vi "DOCK_MAIN_choose_batch_to_reload.vi"(8 "error_in":errorcluster) -> (0 "error_out":errorcluster, 1 "declared_size":u16, 2 "batch_code":string, 3 "batch_ID":string, 5 "Canceled?":bool=TRUE)   [LabVIEW 2019]
uses:
  FGV/SQL_connection/FGV_DOCK_SQL_connection.ctl
  _misc/AULocalize/SubVIs/Get Localized Phrase Compact Interface 1D.vi
  _misc/AULocalize/SubVIs/RegisterVI.vi
panel:
  in  "columns_filter":i32(listbox)
  in  "reload":bool
  in  "cancel":bool
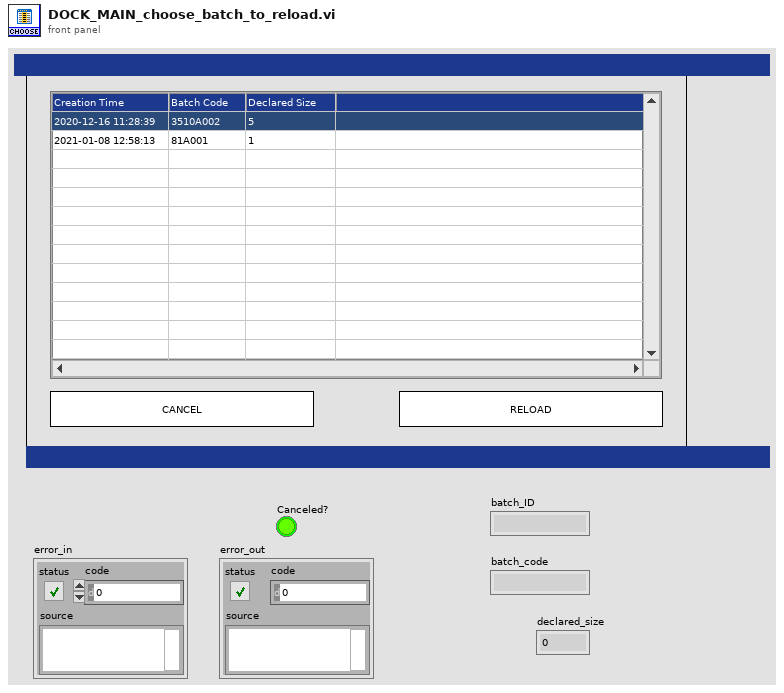
[diagram p1: front panel]
types:
  T1 = typedef "FGV_DOCK_SQL_connection.ctl" = enum16{"initialize", "connect", "read_tables", "read_columns", "SELECT", "INSERT", "UPDATE", "DELETE", "EXEC + headers", "EXEC", "TRANSACTION", "connection_active?", "disconnect"}
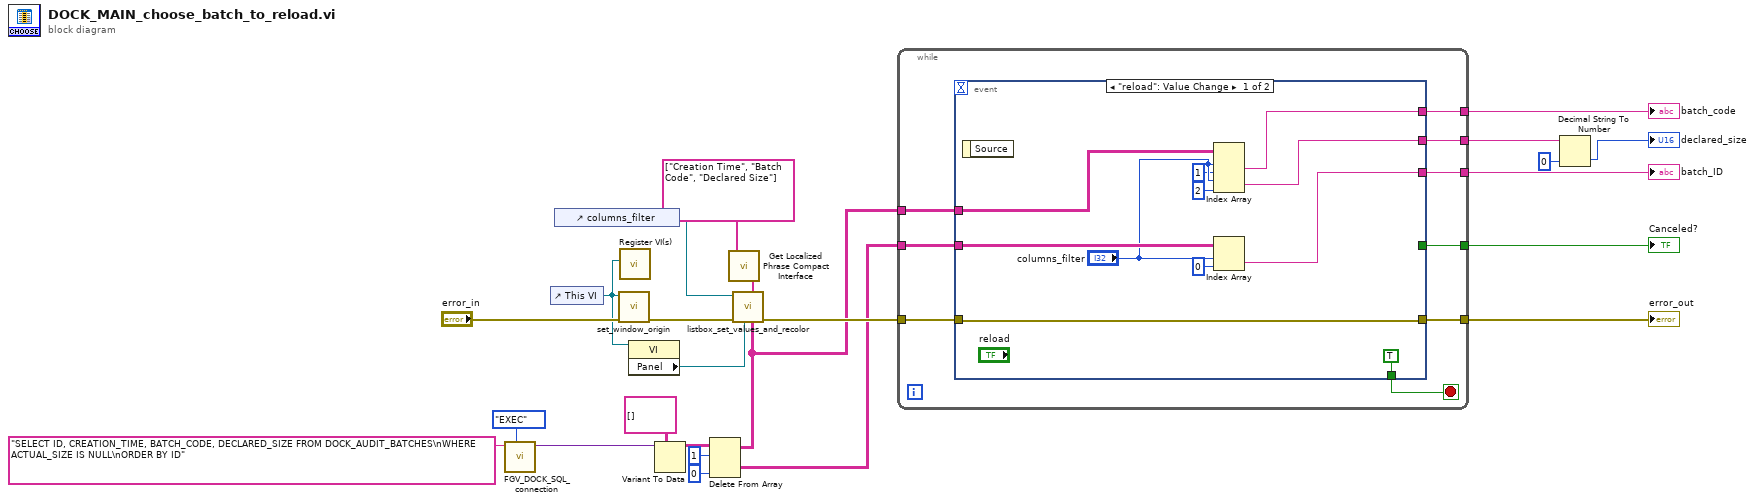
[diagram p0: block diagram]
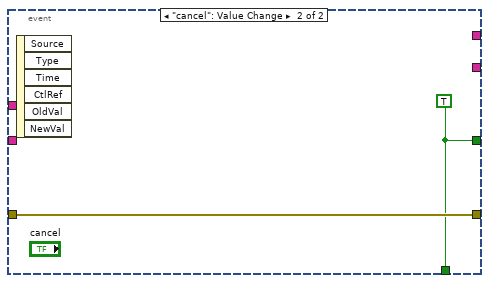
[diagram p2: hidden frame]
diagram:
  n1 = call "FGV_DOCK_SQL_connection.vi"("options"=FGV_DOCK_SQL_connection."EXEC", "SQL_statement"="SELECT ID, CREATION_TIME, BATCH_CODE, DECLARED_SIZE FROM DOCK_AUDIT_BATCHES\nWHERE ACTUAL_SIZE IS NULL\nORDER BY ID") -> ("SQL_result"=w13:variant)  [unwired: 5 in, 4 out]
  n2 = control-ref of="This VI"() -> (w2:refnum<vi>)
  n3 = control-ref of="columns_filter"() -> (w20:refnum<vi>)
  n4 = call "set_window_origin.vi"("error_in"="error_in", "this_vi_reference"=w2) -> ("error_out"=w22:errorcluster)  [unwired: 9 in]
  n5 = call-poly "Register VI(s).vi"("VI Ref"=w2) -> ()  [unwired: 9 in, 2 out]
  n6 = property class="VI"(reference=w2) -> ("Panel"=w19:refnum<vi>)  [unwired: 1 in, 2 out]
  n7 = Variant To Data(type=string[][] [], Variant=w13) -> (data=w12:string[][])  [unwired: 1 in, 1 out]
  n8 = Delete From Array(array=w12, length=1, index (col)=0 ("disabled index (col)")) -> (deleted portion=w9:string[][], array with subset deleted=w7:string[][])  [unwired: 1 in]
  n9 = call-poly "Get Localized Phrase Compact Interface.vi"("Key"=string[] ["Creation Time", "Batch Code", "Declared Size"] ("column_names")) -> ("Translated Phrase"=w1:string[])
  n10 = call "listbox_set_values_and_recolor.vi"("item_names"=w7, "front_panel_reference"=w19, "column_names"=w1, "error_in"=w22, "multicolumn_listbox_reference_in"=w20) -> ("error_out"=w21:errorcluster)  [unwired: 5 in, 1 out]
  n11 = while {
    tunnel: w21 -> [w33]
    tunnel: [w32] -> w24
    tunnel: [w30] -> w17
    tunnel: w9 -> [w29]
    tunnel: [w28] -> w8
    tunnel: w7 -> [w27]
    tunnel: [w26] -> w6
    tunnel: [w25] -> w4
    stop <- w31 stop-if-true
    n12 = event shown="[0] \"reload\": Value Change" {
      selector: _ -> [_ _]
      dyn-events: _ -> [_ _]
      timeout: _ -> [_ _]
      tunnel: w33 -> [w44 w46]
      tunnel: [w44 w46] -> w32
      tunnel: [TRUE w45] -> w31
      tunnel: [_ w45] -> w30
      tunnel: w29 -> [w42 _]
      tunnel: [w40 _] -> w28
      tunnel: w27 -> [w39 _]
      tunnel: [w35 _] -> w26
      tunnel: [w34 _] -> w25
      event "reload": Value Change {
        n13 = event-data() -> ()  [unwired: 1 in, 1 out]
        n14 = Index Array(array=w39, index (row) #1="columns_filter", index (col) #1=1 ("disabled index (col)"), index (row) #2="columns_filter", index (col) #2=2 ("disabled index (col)")) -> (element #1=w35:string, element #2=w34:string)
        n15 = Index Array(array=w42, index (row)="columns_filter", index (col)=0 ("disabled index (col)")) -> (element=w40:string)
      }
      event "cancel": Value Change {
        w45 = TRUE
        n16 = event-data() -> ()  [unwired: 1 in, 6 out]
      }
    }
  }
  "error_out" <- w24
  "Canceled?" <- w17
  "batch_ID" <- w8
  "batch_code" <- w6
  n17 = Decimal String To Number(string=w4, default (0L)=u16 0 ("default (0 I32)")) -> (number=→"declared_size":u16)  [unwired: 1 in, 1 out]
